vi "Delete.vi"(0 "reference in":refnum<class "CustomersBase.lvclass">, 1 "Customer":string, 5 "error in (no error)":errorcluster) -> (14 "reference out":refnum<class "CustomersBase.lvclass">, 19 "error out":errorcluster)   [LabVIEW 2020, in "CustomersBase.lvclass"]
uses:
  CustomersBase.lvclass
  DataObject_class/DataObject.lvclass
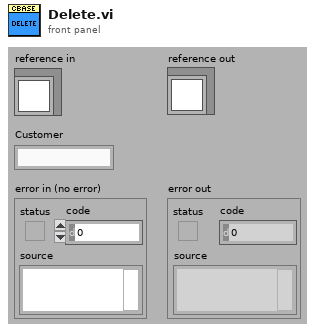
[diagram p1: front panel]
types:
  T1 = typedef "CustomersBase.lvclass/ObjectAttributes.ctl" = cluster{"_dataObject":refnum<class "DataObject.lvclass">, "Group":string}
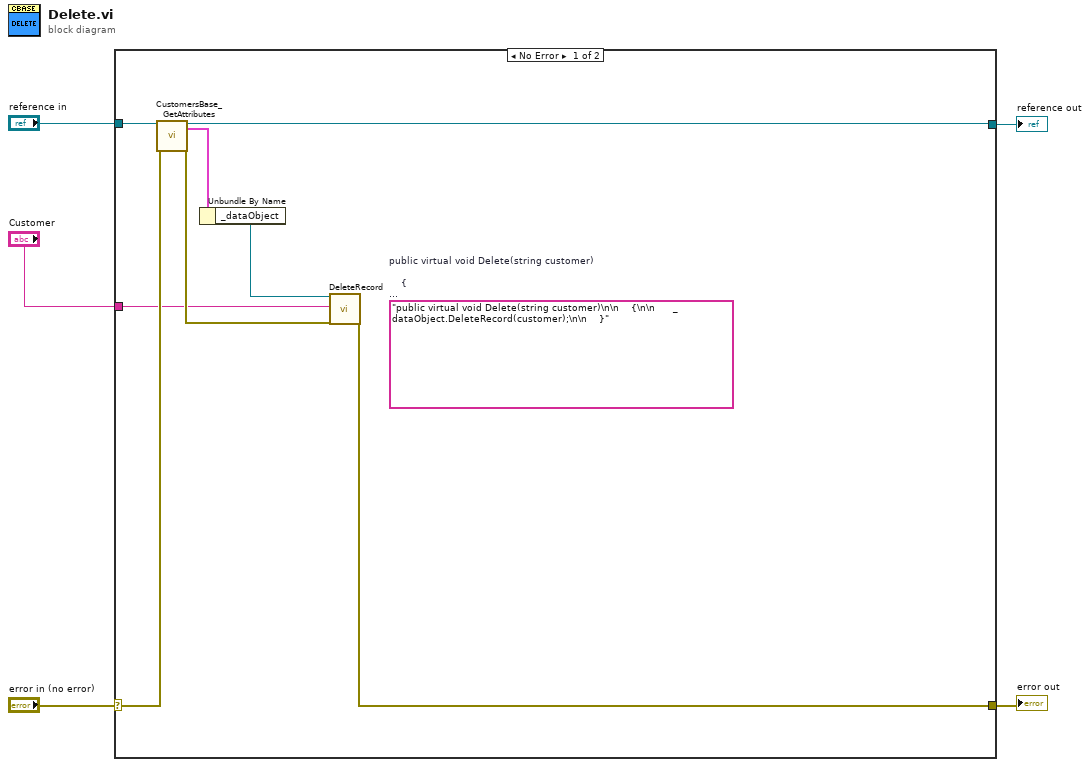
[diagram p0: block diagram]
diagram:
  n1 = case shown="No Error" "error in (no error)" {
    selector: "error in (no error)" -> [w12 w15]
    tunnel: [w7 w15] -> w4
    tunnel: [w10 w14] -> w2
    tunnel: "reference in" -> [w13 w14]
    tunnel: "Customer" -> [w6 _]
    frame No Error {
      (unwired) "public virtual void Delete(string customer)\n\n    {\n\n      _dataObject.DeleteRecord(customer);\n\n    }"  # public virtual void Delete(string customer)      {        _dataObject.DeleteRecord(customer);      }
      n2 = call "CustomersBase_GetAttributes.vi"("reference in"=w13, "error in (no error)"=w12) -> ("reference out"=w10:refnum<class "CustomersBase.lvclass">, "Data"=w11:T1, "error out"=w8:errorcluster)  [unwired: 14 in, 1 out]
      n3 = Unbundle By Name(w11) -> ("_dataObject"=w9:refnum<class "DataObject.lvclass">)
      n4 = call-dynamic "DeleteRecord.vi"("reference in"=w9, "Record"=w6, "error in (no error)"=w8) -> ("error out"=w7:errorcluster)  [unwired: 15 in, 1 out]
    }
    frame Error {
    }
  }
  "error out" <- w4
  "reference out" <- w2
